vi "Initialize.vi"(8 "error in (no error)":errorcluster, 10 "Instrument Refnum in":refnum<visa-resource-name>, 11 "Simulate in":refnum<class "Simulated DMM.lvclass">) -> (0 "error out":errorcluster, 2 "Result Text":string="PCI-4070 has been initialized", 3 "Simulate out":refnum<class "Simulated DMM.lvclass">)   [LabVIEW 2012, in "Simulated DMM.lvclass"]
uses:
  Simulated DMM.lvclass
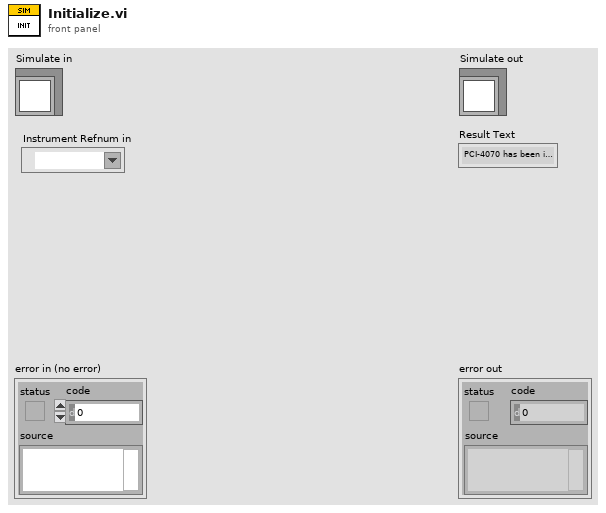
[diagram p1: front panel]
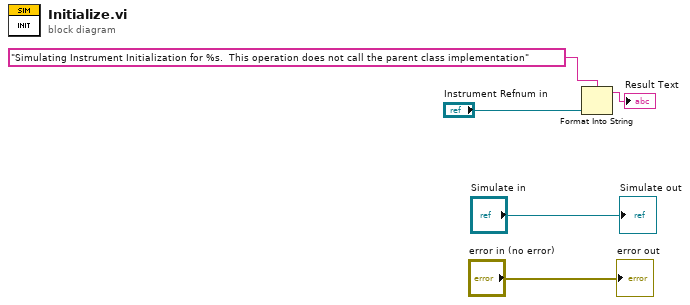
[diagram p0: block diagram]
diagram:
  n1 = Format Into String(format string="Simulating Instrument Initialization for %s.  This operation does not call the parent class implementation" ("message"), "Instrument Refnum in") -> (resulting string=→"Result Text":string)  [unwired: 2 in, 1 out]
  "error out" <- "error in (no error)"
  "Simulate out" <- "Simulate in"
